vi "selfTest.vi"(0 "NInstrSim":refnum<class "NInstrSim.lvclass">, 5 "error in (no error)":errorcluster) -> (14 "dup NInstrSim":refnum<class "NInstrSim.lvclass">, 16 "passed?":bool, 17 "resultCode":i32, 18 "resultMessage":string, 19 "error out":errorcluster)   [LabVIEW 2009, in "HB_Device_Examples.lvlib" / "NInstrSim.lvclass"]
doc: "This VI runs the instrument's self test routine and returns the test results."
uses:
  NInstrSim.lvclass
  NInstrSim.lvclass/NInstrSim.ctl
  non_GPL/instr.lib/NI Instrument Simulator/NI Instrument Simulator.lvlib
  lib.lib/HGF_LVC/HGF_DeviceBaseClasses/HGF_VISADevice/HGF_VISADevice.lvclass
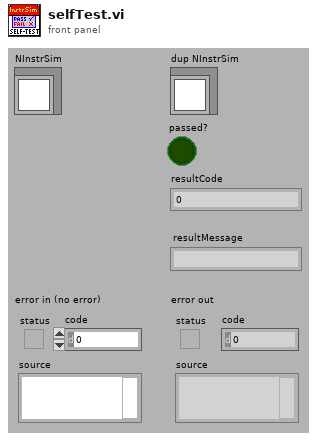
[diagram p1: front panel]
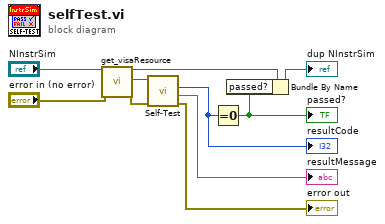
[diagram p0: block diagram]
diagram:
  n1 = call "get_visaResource.vi"("HGF_VISADevice"="NInstrSim", "error in (no error)"="error in (no error)") -> ("dup HGF_VISADevice"=w3:refnum<class "NInstrSim.lvclass">, "VISA Resource Name"=w7:refnum<visa-resource-name>, "error out"=w8:errorcluster)  [unwired: 15 out]
  n2 = call "Self-Test.vi"("error in (no error)"=w8, "VISA resource name"=w7) -> ("error out"=→"error out":errorcluster, "Self-Test Result Message"=→"resultMessage":string, "Self-Test Result Code"=w4:i32)  [unwired: 7 out]
  "resultCode" <- w4
  n3 = Equal To 0?(x=w4) -> (x = 0?=w1:bool)
  "passed?" <- w1
  n4 = Bundle By Name(cluster=w3, "passed?"=w1) -> (→"dup NInstrSim":refnum<class "NInstrSim.lvclass">)
